vi "PIDdebuger.vi"() -> ()   [LabVIEW 2015]
doc: "的发给伺服"
uses:
  <vilib>/Platform/browser.llb/Open URL in Default Browser (string).vi
  lib/pcomm/PCOMM.DLL
  lib/pcomm/PCOMM.lvlib
panel:
  in  "刷新按钮":bool
  out "字符串 3":string="PID目标值"
  out "字符串 2":string="串口设置"
  in  "串口号":i32(ring)=1 items=["COM1 通信端口 (COM1)"=1, "COM2 ELTIMA Virtual Serial Port (COM2->COM3)"=2, "COM3 ELTIMA Virtual Serial Port (COM3->COM2)"=3, "COM8 USB-SERIAL CH340 (COM8)"=8]
  in  "波特率":i32(ring)=16 items=["1800"=8, "2400"=9, "4800"=10, "7200"=11, "9600"=12, "19200"=13, "38400"=14, "57600"=15, "115200"=16, "230400"=17, "460800"=18, "921600"=19]
  in  "数据比特":i32(ring)=3 caption="数据位" items=["5", "6", "7", "8"]
  in  "停止位":i32(ring) items=["1"=0, "2"=4]
  in  "奇偶校验":i32(ring) caption="校   验" items=["None"=0, "Odd"=8, "Even"=24, "Mark"=40, "Space"=56]
  in  "打开/关闭串口":bool
  in  "清除图表":bool
  in  "启动电机":bool
  in  "复位":bool
  out "目标值_s":i32
  out "反馈值":i32
  out "波形图表":cluster{"Value":i32, i32, i32, i32}(graph)
  in  "发送PID":bool
  in  "目标值":i32
  in  "D":sgl
  in  "I":sgl
  in  "P":sgl
  in  "发送目标值":bool
  # "目前适用的例程: \nYS-F4Pro的有刷和无刷相关例程\nYS-H7Multi的步进电机相关例程\nYS-H7Multi的有刷电机相关例程"
  # "操作提示：\n1. 先关闭串口,再拖动图像。\n2.可在右边绘图控制区改变曲线显示样式。\n3.在绘图区右击可以导出图像到excel,剪切板。"
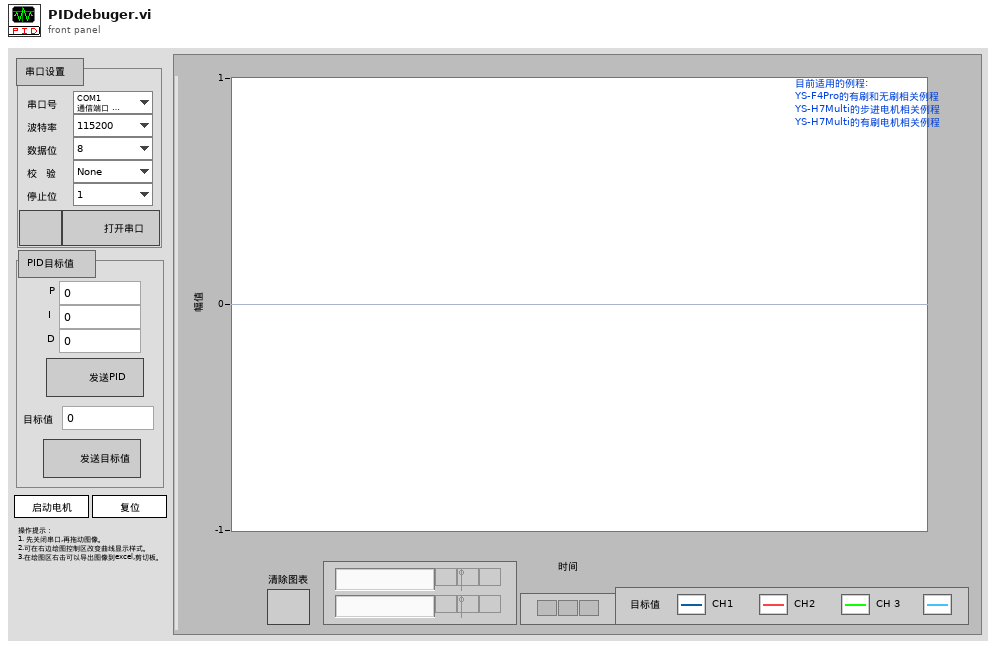
[diagram p1: front panel]
types:
  T1 = enum8{"Enabled", "Disabled", "Disabled and Grayed Out"}
  T2 = typedef "LVRectTypeDef.ctl" = cluster{"Left":i16, "Top":i16, "Right":i16, "Bottom":i16}
  T3 = typedef "LVPointTypeDef.ctl" = cluster{"Horizontal":i16, "Vertical":i16}
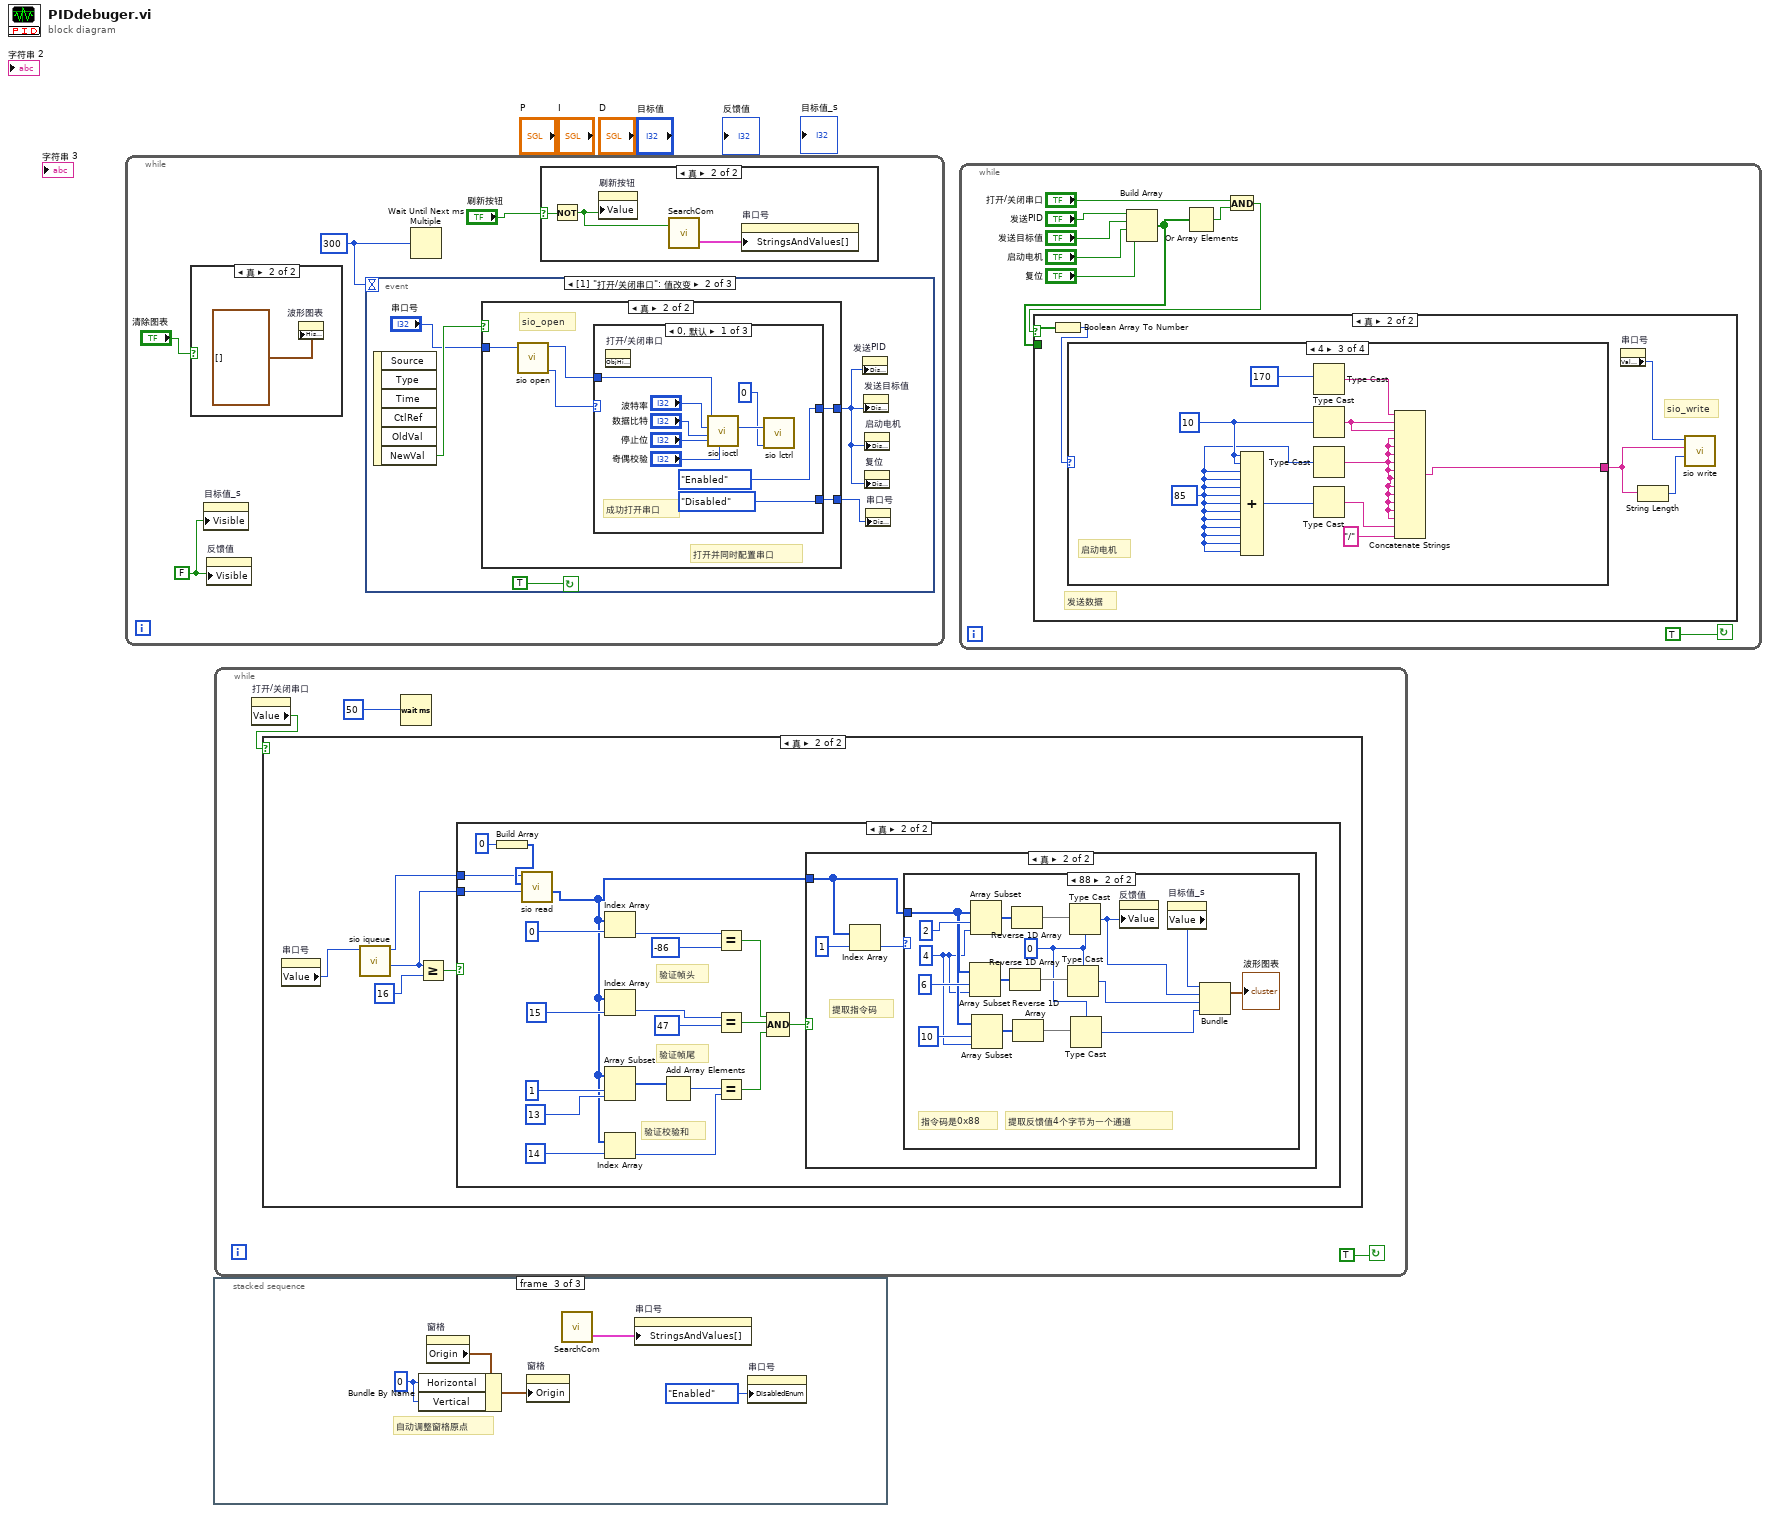
[diagram p0: block diagram]
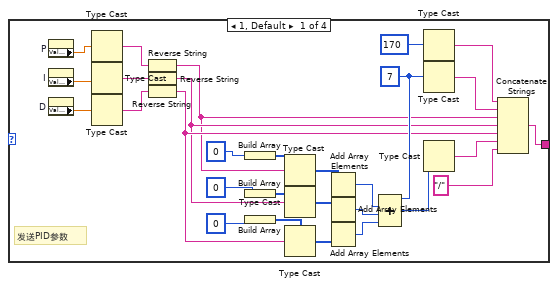
[diagram p3: hidden frame]
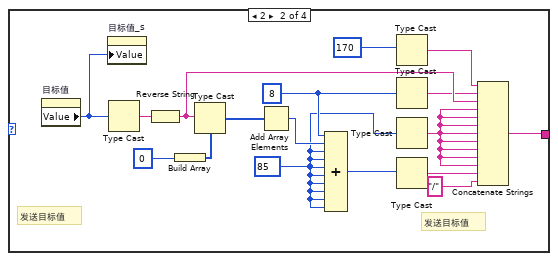
[diagram p4: hidden frame]
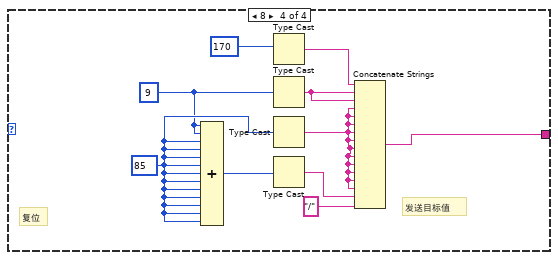
[diagram p5: hidden frame]
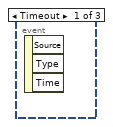
[diagram p8: hidden frame]
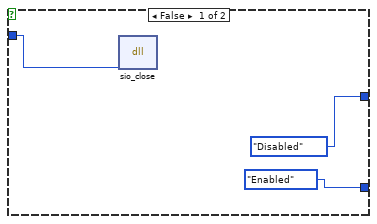
[diagram p9: hidden frame]
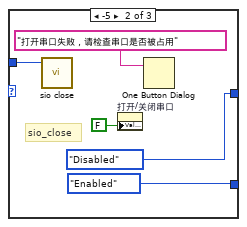
[diagram p10: hidden frame]
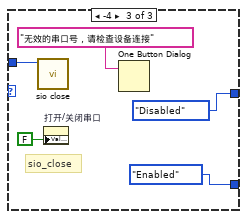
[diagram p11: hidden frame]
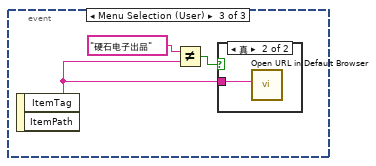
[diagram p12: hidden frame]
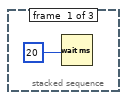
[diagram p14: hidden frame]
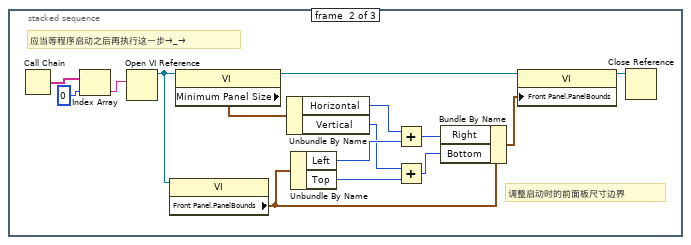
[diagram p15: hidden frame]
diagram:
  n1 = while {
    stop <- TRUE continue-if-true
    w2 = FALSE
    w4 = 300
    n2 = case shown="真" "清除图表" {
      frame False {
      }
      frame True {
        n3 = property on="波形图表" class="WFChart (严格)"("History Data"=cluster{i32, i32, i32, i32}[] []) -> ()  [unwired: 2 in, 2 out]
      }
    }
    n4 = property on="目标值_s" class="DigNum (严格)"("Visible"=w2) -> ()  [unwired: 2 in, 2 out]
    n5 = property on="反馈值" class="DigNum (严格)"("Visible"=w2) -> ()  [unwired: 2 in, 2 out]
    n6 = event shown="[1] \"打开/关闭串口\": 值改变" {
      selector: _ -> [_ _ _]
      dyn-events: _ -> [_ _ _]
      timeout: w4 -> [_ _ _]
      event Timeout {
        n7 = event-data() -> ()  [unwired: 1 in, 3 out]
      }
      event "打开/关闭串口": Value Change {
        n8 = event-data() -> ("NewVal"=w13:bool)  [unwired: 1 in, 5 out]
        n9 = case shown="真" w13 {
          tunnel: "串口号" -> [w16 w17]
          tunnel: [T1."Disabled" w19] -> w11
          tunnel: [T1."Enabled" w18] -> w10
          frame False {
            n10 = dll-call lib="PTH2Yabs EDesktopLabview串口助手串口助手2.0Ing10_v3.2.0libpcommPCOMM.*" fn="sio_close"("port"=w16) -> ()  [unwired: 5 in, 2 out]
          }
          frame True {
            # "sio_open"
            # "打开并同时配置串口"
            n11 = call "sio open.vi"("port"=w17) -> ("port"=w20:i32, "Status"=w21:i32)  [unwired: 6 in]
            n12 = case shown="0, 默认" w21 {
              tunnel: w20 -> [w26 w31 w36]
              tunnel: [T1."Enabled" T1."Disabled" T1."Disabled"] -> w19
              tunnel: [T1."Disabled" T1."Enabled" T1."Enabled"] -> w18
              frame 0, Default {
                # "成功打开串口"
                n13 = invoke on="打开/关闭串口" class="Bool (严格)" method="ObjHighlight"() -> ()  [unwired: 3 in, 3 out]
                n14 = call "sio ioctl.vi"("parity"="奇偶校验", "stop bits"="停止位", "data bits"="数据比特", "baud"="波特率", "port"=w26) -> ("port"=w23:i32)  [unwired: 5 in, 1 out]
                n15 = call "sio lctrl.vi"("mode"=0, "port"=w23) -> ()  [unwired: 8 in, 2 out]
              }
              frame -5 {
                # "sio_close"
                n16 = call "sio close.vi"("port"=w31) -> ()  [unwired: 9 in, 2 out]
                n17 = property on="打开/关闭串口" class="Bool (严格)"("Value"=FALSE) -> ()  [unwired: 2 in, 2 out]
                n18 = One Button Dialog(message="打开串口失败，请检查串口是否被占用") -> ()  [unwired: 1 in, 1 out]
              }
              frame -4 {
                # "sio_close"
                n19 = call "sio close.vi"("port"=w36) -> ()  [unwired: 9 in, 2 out]
                n20 = property on="打开/关闭串口" class="Bool (严格)"("Value"=FALSE) -> ()  [unwired: 2 in, 2 out]
                n21 = One Button Dialog(message="无效的串口号，请检查设备连接") -> ()  [unwired: 1 in, 1 out]
              }
            }
          }
        }
        n22 = property on="发送PID" class="Bool"("DisabledEnum"=w11) -> ()  [unwired: 2 in, 2 out]
        n23 = property on="发送目标值" class="Bool"("DisabledEnum"=w11) -> ()  [unwired: 2 in, 2 out]
        n24 = property on="启动电机" class="Bool"("DisabledEnum"=w11) -> ()  [unwired: 2 in, 2 out]
        n25 = property on="复位" class="Bool"("DisabledEnum"=w11) -> ()  [unwired: 2 in, 2 out]
        n26 = property on="串口号" class="Ring (严格)"("DisabledEnum"=w10) -> ()  [unwired: 2 in, 2 out]
      }
      event Menu Selection (User) {
        n27 = event-data() -> ("ItemTag"=w41:string)  [unwired: 1 in, 1 out]
        n28 = Not Equal?(x="硬石电子出品", y=w41) -> (x != y?=w42:bool)
        n29 = case shown="真" w42 {
          tunnel: w41 -> [_ w44]
          frame False {
          }
          frame True {
            n30 = call-poly <vilib>:"Open URL in Default Browser.vi"("URL"=w44) -> ()  [unwired: 5 in, 2 out]
          }
        }
      }
    }
    n31 = Wait Until Next ms Multiple(millisecond multiple=w4) -> ()  [unwired: 1 out]
    n32 = case shown="真" "刷新按钮" {
      selector: "刷新按钮" -> [_ w7]
      frame False {
      }
      frame True {
        n33 = Not(x=w7) -> (.not. x?=w6:bool)
        n34 = property on="刷新按钮" class="Bool (严格)"("Value"=w6) -> ()  [unwired: 2 in, 2 out]
        n35 = call "SearchCom.vi"("使用注册表？"=w6) -> ("下拉列表项"=w8:cluster{"String":string, "Value":i32}[])  [unwired: 2 in]
        n36 = property on="串口号" class="Ring (严格)"("StringsAndValues[]"=w8) -> ()  [unwired: 2 in, 2 out]
      }
    }
  }
  n37 = stacked-sequence {
    frame #0 {
      n38 = Wait (ms)(milliseconds to wait=u32 20) -> ()  [unwired: 1 out]
    }
    frame #1 {
      # "调整启动时的前面板尺寸边界"
      # "应当等程序启动之后再执行这一步→_→"
      n39 = Call Chain ("调用链")() -> (call chain=w48:string[])
      n40 = Index Array(array=w48, index=0) -> (element=w46:string)
      n41 = Open VI Reference(vi path=w46) -> (vi reference=w58:refnum<vi>)  [unwired: 1 in, 5 out]
      n42 = property class="VI"(reference=w58) -> ("Front Panel.PanelBounds"=w55:T2)  [unwired: 1 in, 2 out]
      n43 = property class="VI"(reference=w58) -> (reference out=w59:refnum<vi>, "Minimum Panel Size"=w49:T3)  [unwired: 1 in, 1 out]
      n44 = Unbundle By Name(w49) -> ("Horizontal"=w56:i16, "Vertical"=w53:i16)
      n45 = Unbundle By Name(w55) -> ("Left"=w57:i16, "Top"=w52:i16)
      n46 = Add(x=w56, y=w57) -> (x+y=w54:i16)
      n47 = Add(x=w53, y=w52) -> (x+y=w51:i16)
      n48 = Bundle By Name(cluster=w55, "Right"=w54, "Bottom"=w51) -> (w50:T2)
      n49 = property class="VI"(reference=w59, "Front Panel.PanelBounds"=w50) -> (reference out=w60:refnum<vi>)  [unwired: 1 in, 1 out]
      n50 = Close Reference(reference=w60) -> ()  [unwired: 1 in, 1 out]
    }
    frame #2 {
      w65 = i16 0
      # "自动调整窗格原点"
      n51 = property on="窗格" class="Pane"() -> ("Origin"=w64:T3)  [unwired: 2 in, 2 out]
      n52 = Bundle By Name(cluster=w64, "Horizontal"=w65, "Vertical"=w65) -> (w63:T3)
      n53 = property on="窗格" class="Pane"("Origin"=w63) -> ()  [unwired: 2 in, 2 out]
      n54 = call "SearchCom.vi"() -> ("下拉列表项"=w61:cluster{"String":string, "Value":i32}[])  [unwired: 3 in]
      n55 = property on="串口号" class="Ring (严格)"("StringsAndValues[]"=w61) -> ()  [unwired: 2 in, 2 out]
      n56 = property on="串口号" class="Ring (严格)"("DisabledEnum"=T1."Enabled" ("禁用")) -> ()  [unwired: 2 in, 2 out]
    }
  }
  n57 = while {
    stop <- TRUE continue-if-true
    n58 = property on="打开/关闭串口" class="Bool (严格)"() -> ("Value"=w66:bool)  [unwired: 2 in, 2 out]
    n59 = case shown="真" w66 {
      frame False {
      }
      frame True {
        n60 = property on="串口号" class="Ring (严格)"() -> ("Value"=w70:i32)  [unwired: 2 in, 2 out]
        n61 = call "sio iqueue.vi"("port"=w70) -> ("len"=w71:i32, "port"=w69:i32)  [unwired: 8 in, 1 out]
        n62 = Greater Or Equal?(x=w71, y=16) -> (x >= y?=w72:bool)
        n63 = case shown="真" w72 {
          tunnel: w71 -> [_ w76]
          tunnel: w69 -> [_ w75]
          frame False {
          }
          frame True {
            # "验证帧尾"
            # "验证校验和"
            # "验证帧头"
            n64 = Build Array(i8 0) -> (w77:i8[])
            n65 = call "sio read.vi"("len"=w76, "buf"=w77, "port"=w75) -> ("buf out"=w74:i8[])  [unwired: 4 in, 3 out]
            n66 = Index Array(array=w74, index=0) -> (element=w92:i8)
            n67 = Index Array(array=w74, index=15) -> (element=w89:i8)
            n68 = Array Subset(array=w74, index=1, length=13) -> (w82:i8[])
            n69 = Index Array(array=w74, index=14) -> (element=w85:i8)
            n70 = Add Array Elements(numeric array=w82) -> (sum=w84:i8)
            n71 = Equal?(x=w92, y=i8 -86) -> (x = y?=w90:bool)
            n72 = Equal?(x=w89, y=i8 47) -> (x = y?=w86:bool)
            n73 = Equal?(x=w84, y=w85) -> (x = y?=w80:bool)
            n74 = Compound Arithmetic op=AND ("复合运算")(w90, w86, w80) -> (w94:bool)
            n75 = case shown="真" w94 {
              tunnel: w74 -> [_ w95]
              frame False {
              }
              frame True {
                # "提取指令码"
                n76 = Index Array(array=w95, index=1) -> (element=w96:i8)
                n77 = case shown="88" w96 {
                  tunnel: w95 -> [_ w107]
                  frame Default {
                    # "指令码0x00,无效"
                  }
                  frame -120 {
                    w98 = 0
                    w106 = 4
                    # "指令码是0x88"
                    # "提取反馈值4个字节为一个通道"
                    n78 = Array Subset(array=w107, index=6, length=w106) -> (w103:i8[])
                    n79 = Array Subset(array=w107, index=2, length=w106) -> (w113:i8[])
                    n80 = Array Subset(array=w107, index=10, length=w106) -> (w100:i8[])
                    n81 = Reverse 1D Array(array=w103) -> (reversed array=w105:i8[])
                    n82 = Reverse 1D Array(array=w113) -> (reversed array=w112:i8[])
                    n83 = Reverse 1D Array(array=w100) -> (reversed array=w101:i8[])
                    n84 = Type Cast(type=w98, x=w105) -> (*(type *) &x=w102:i32)
                    n85 = Type Cast(type=w98, x=w112) -> (*(type *) &x=w110:i32)
                    n86 = Type Cast(type=w98, x=w101) -> (*(type *) &x=w99:i32)
                    n87 = property on="反馈值" class="DigNum (严格)"("Value"=w110) -> ()  [unwired: 2 in, 2 out]
                    n88 = property on="目标值_s" class="DigNum (严格)"() -> ("Value"=w111:i32)  [unwired: 2 in, 2 out]
                    n89 = Bundle("Value"=w111, w110, w102, w99) -> (→"波形图表":cluster{"Value":i32, i32, i32, i32})  [unwired: 1 in]
                  }
                }
              }
            }
          }
        }
      }
    }
    n90 = Wait (ms)(milliseconds to wait=u32 50) -> ()  [unwired: 1 out]
  }
  n91 = while {
    stop <- TRUE continue-if-true
    n92 = Build Array("发送PID", "发送目标值", "启动电机", "复位") -> (w118:bool[])
    n93 = Or Array Elements(Boolean array=w118) -> (logical OR=w117:bool)
    n94 = And ("与")(x="打开/关闭串口", y=w117) -> (x .and. y?=w116:bool)
    n95 = case shown="真" w116 {
      tunnel: w118 -> [_ w128]
      frame False {
      }
      frame True {
        # "sio_write"
        # "发送数据"
        n96 = Boolean Array To Number(Boolean array=w128) -> (number=w127:u32)
        n97 = case shown="4" w127 {
          tunnel: [w129 w158 w176 w185] -> w125
          frame 1, Default {
            w133 = u8 7
            # "发送PID参数"
            n98 = property on="P" class="DigNum (严格)"() -> ("Value"=w143:sgl)  [unwired: 2 in, 2 out]
            n99 = property on="I" class="DigNum (严格)"() -> ("Value"=w144:sgl)  [unwired: 2 in, 2 out]
            n100 = property on="D" class="DigNum (严格)"() -> ("Value"=w150:sgl)  [unwired: 2 in, 2 out]
            n101 = Type Cast(x=w143) -> (*(type *) &x=w155:string)  [unwired: 1 in]
            n102 = Type Cast(x=w144) -> (*(type *) &x=w156:string)  [unwired: 1 in]
            n103 = Type Cast(x=w150) -> (*(type *) &x=w157:string)  [unwired: 1 in]
            n104 = Reverse String(1:w155) -> (0:w130:string)
            n105 = Reverse String(1:w156) -> (0:w131:string)
            n106 = Reverse String(1:w157) -> (0:w132:string)
            n107 = Build Array(u8 0) -> (w140:u8[])
            n108 = Build Array(u8 0) -> (w145:u8[])
            n109 = Build Array(u8 0) -> (w134:u8[])
            n110 = Type Cast(type=w140, x=w130) -> (*(type *) &x=w141:u8[])
            n111 = Type Cast(type=w145, x=w131) -> (*(type *) &x=w147:u8[])
            n112 = Type Cast(type=w134, x=w132) -> (*(type *) &x=w151:u8[])
            n113 = Add Array Elements(numeric array=w141) -> (sum=w142:u8)
            n114 = Add Array Elements(numeric array=w147) -> (sum=w148:u8)
            n115 = Add Array Elements(numeric array=w151) -> (sum=w152:u8)
            n116 = Compound Arithmetic op=ADD(w133, w142, w148, w152) -> (w136:u8)
            n117 = Type Cast(x=u8 170) -> (*(type *) &x=w137:string)  [unwired: 1 in]
            n118 = Type Cast(x=w133) -> (*(type *) &x=w138:string)  [unwired: 1 in]
            n119 = Type Cast(x=w136) -> (*(type *) &x=w153:string)  [unwired: 1 in]
            n120 = Concatenate Strings(w137, w138, w130, w131, w132, w153, "/") -> (w129:string)
          }
          frame 2 {
            w159 = u8 85
            w164 = u8 8
            # "发送目标值"
            # "发送目标值"
            n121 = property on="目标值" class="DigNum (严格)"() -> ("Value"=w174:i32)  [unwired: 2 in, 2 out]
            n122 = property on="目标值_s" class="DigNum (严格)"("Value"=w174) -> ()  [unwired: 2 in, 2 out]
            n123 = Type Cast(x=w174) -> (*(type *) &x=w172:string)  [unwired: 1 in]
            n124 = Reverse String(1:w172) -> (0:w173:string)
            n125 = Build Array(u8 0) -> (w169:u8[])
            n126 = Type Cast(type=w169, x=w173) -> (*(type *) &x=w170:u8[])
            n127 = Add Array Elements(numeric array=w170) -> (sum=w171:u8)
            n128 = Compound Arithmetic op=ADD(w164, w171, w159, w159, w159, w159, w159, w159, w159, w159) -> (w161:u8)
            n129 = Type Cast(x=u8 170) -> (*(type *) &x=w162:string)  [unwired: 1 in]
            n130 = Type Cast(x=w164) -> (*(type *) &x=w163:string)  [unwired: 1 in]
            n131 = Type Cast(x=w159) -> (*(type *) &x=w166:string)  [unwired: 1 in]
            n132 = Type Cast(x=w161) -> (*(type *) &x=w167:string)  [unwired: 1 in]
            n133 = Concatenate Strings(w162, w163, w173, w166, w166, w166, w166, w166, w166, w166, w166, w167, "/") -> (w158:string)
          }
          frame 4 {
            w175 = u8 85
            w184 = u8 10
            # "启动电机"
            n134 = Compound Arithmetic op=unknown(w184, w184, w175, w175, w175, w175, w175, w175, w175, w175, w175, w175, w175) -> (w178:u8)
            n135 = Type Cast(x=u8 170) -> (*(type *) &x=w179:string)  [unwired: 1 in]
            n136 = Type Cast(x=w184) -> (*(type *) &x=w180:string)  [unwired: 1 in]
            n137 = Type Cast(x=w175) -> (*(type *) &x=w183:string)  [unwired: 1 in]
            n138 = Type Cast(x=w178) -> (*(type *) &x=w182:string)  [unwired: 1 in]
            n139 = Concatenate Strings(w179, w180, w180, w183, w183, w183, w183, w183, w183, w183, w183, w183, w183, w183, w182, "/") -> (w176:string)
          }
          frame 8 {
            w187 = u8 85
            w186 = u8 9
            # "发送目标值"
            # "复位"
            n140 = Compound Arithmetic op=unknown(w186, w186, w187, w187, w187, w187, w187, w187, w187, w187, w187, w187, w187) -> (w193:u8)
            n141 = Type Cast(x=u8 170) -> (*(type *) &x=w192:string)  [unwired: 1 in]
            n142 = Type Cast(x=w186) -> (*(type *) &x=w191:string)  [unwired: 1 in]
            n143 = Type Cast(x=w187) -> (*(type *) &x=w188:string)  [unwired: 1 in]
            n144 = Type Cast(x=w193) -> (*(type *) &x=w189:string)  [unwired: 1 in]
            n145 = Concatenate Strings(w192, w191, w191, w188, w188, w188, w188, w188, w188, w188, w188, w188, w188, w188, w189, "/") -> (w185:string)
          }
        }
        n146 = property on="串口号" class="Ring (严格)"() -> ("Value"=w124:i32)  [unwired: 2 in, 2 out]
        n147 = String Length(string=w125) -> (length=w126:i32)
        n148 = call "sio write.vi"("len"=w126, "buf"=w125, "port"=w124) -> ()  [unwired: 6 in, 3 out]
      }
    }
  }
